vi "FGV_OutputHeaderFormat.vi"(7 "Mode":T1, 8 "error in (no error)":errorcluster, 10 "Long Header?":bool=TRUE, 11 "Header On?":bool=TRUE) -> (0 "error out":errorcluster, 2 "Long Header?":bool=TRUE, 3 "Header On?":bool=TRUE)   [LabVIEW 2018, in "OXYGEN.lvlib"]
uses:
  OXYGEN.lvlib
  TypeDefs/Modes_FGV_OutputHeaderFormat.ctl
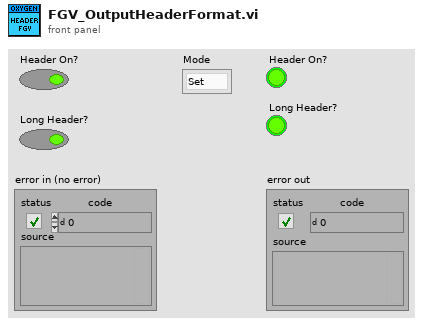
[diagram p1: front panel]
types:
  T1 = typedef "OXYGEN.lvlib/Modes_FGV_OutputHeaderFormat.ctl" = enum16{"Set", "Get"}
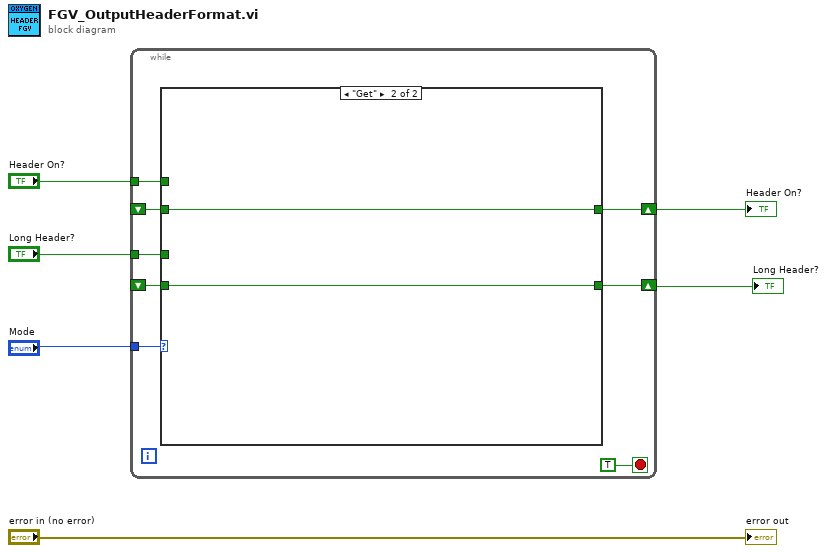
[diagram p0: block diagram]
diagram:
  n1 = while {
    tunnel: "Mode" -> [w14]
    tunnel: "Header On?" -> [w12]
    shift-right: [w11] -> w2
    shift-left: _ -> [w8]
    tunnel: "Long Header?" -> [w10]
    shift-right: [w9] -> w1
    shift-left: _ -> [w7]
    stop <- TRUE stop-if-true
    n2 = case shown="\"Get\"" w14 {
      tunnel: w12 -> [w16 _]
      tunnel: [w16 w18] -> w11
      tunnel: w10 -> [w15 _]
      tunnel: [w15 w17] -> w9
      tunnel: w8 -> [_ w18]
      tunnel: w7 -> [_ w17]
      frame "Set", Default {
      }
      frame "Get" {
      }
    }
  }
  "Long Header?" <- w1
  "Header On?" <- w2
  "error out" <- "error in (no error)"
